vi "Select SubProtocol.vi"(7 "Set?":bool, 8 "error in (no error)":errorcluster, 11 "Connection.WS in":refnum<class "Connection.WS.lvclass">) -> (0 "error out":errorcluster, 3 "Connection.WS out":refnum<class "Connection.WS.lvclass">)   [LabVIEW 2013, in "Connection.WS_GOSPL.lvlib" / "Connection.WS.lvclass"]
uses:
  Connection.WS.lvclass
  Connection.WS.lvclass/Connection.WS.ctl
  Header Fields -- combo.ctl
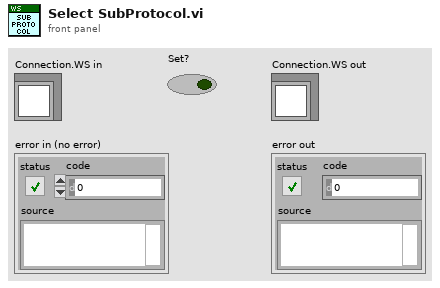
[diagram p1: front panel]
types:
  T1 = typedef "Connection.WS_GOSPL.lvlib/Connection.WS.lvclass/Header Fields -- combo.ctl" = string
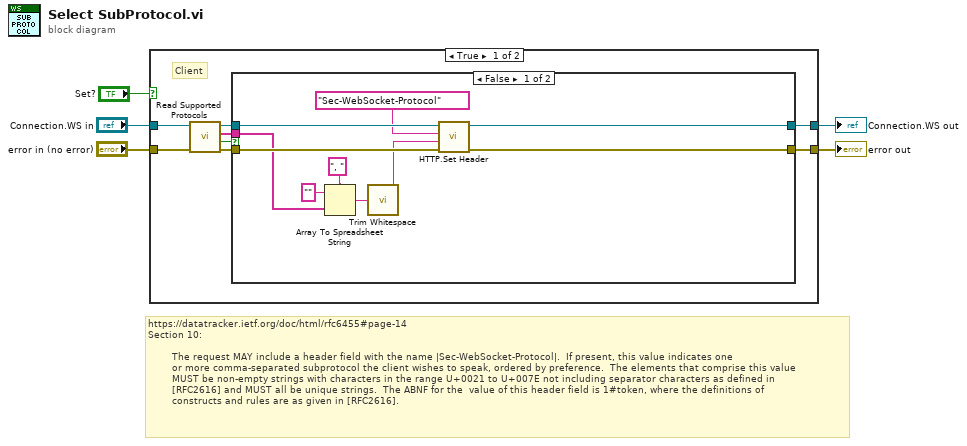
[diagram p0: block diagram]
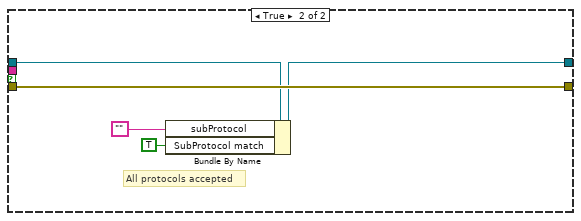
[diagram p2: hidden frame]
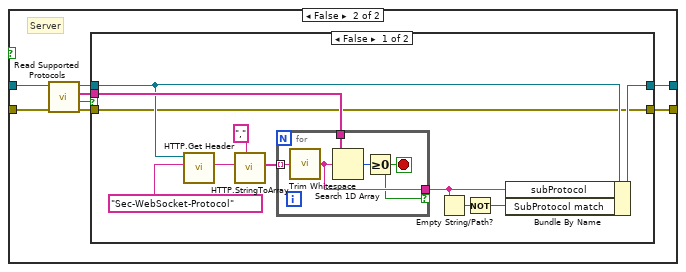
[diagram p3: hidden frame]
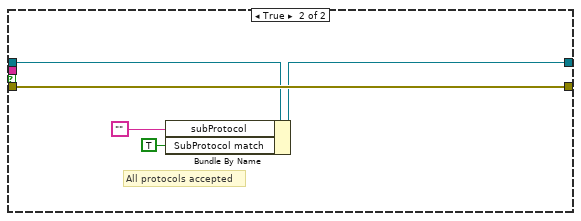
[diagram p4: hidden frame]
diagram:
  # "https://datatracker.ietf.org/doc/html/rfc6455#page-14\nSection 10:\n\n        The request MAY include a header field with the name |Sec-WebSocket-Protocol|.  If present, this value indicates one\n        or more comma-separated subprotocol the client wishes to speak, ordered by preference.  The elements that comprise this value\n        MUST be non-empty strings with characters in the range U+0021 to U+007E not including separator characters as defined in\n        [RFC2616] and MUST all be unique strings.  The ABNF for the  value of this header field is 1#token, where the definitions of\n        constructs and rules are as given in [RFC2616]."
  n1 = case shown="True" "Set?" {
    tunnel: [w11 w34] -> w5
    tunnel: [w10 w33] -> w4
    tunnel: "Connection.WS in" -> [w7 w30]
    tunnel: "error in (no error)" -> [w6 w29]
    frame True {
      # "Client"
      n2 = call "Read Supported Protocols.vi"("error in (no error)"=w6, "Connection.WS in"=w7) -> ("error out"=w12:errorcluster, "All?"=w8:bool, "Supported Protocols"=w13:string[], "Connection.WS out"=w9:refnum<class "Connection.WS.lvclass">)  [unwired: 6 in]
      n3 = case shown="False" w8 {
        tunnel: w9 -> [w23 w26]
        tunnel: [w22 w25] -> w10
        tunnel: [w20 w28] -> w11
        tunnel: w12 -> [w21 w28]
        tunnel: w13 -> [w18 _]
        frame False {
          n4 = Array To Spreadsheet String(delimiter (Tab)=", ", array=w18, 3:"" ("format string")) -> (spreadsheet string=w16:string)
          n5 = call <vilib>:"Trim Whitespace.vi"("string"=w16) -> ("trimmed string"=w14:string)  [unwired: 1 in]
          n6 = call "HTTP.Set Header.vi"("error in (no error)"=w21, "Value"=w14, "Header Name"=T1 "Sec-WebSocket-Protocol", "Connection.WS in"=w23) -> ("error out"=w20:errorcluster, "Connection.WS out"=w22:refnum<class "Connection.WS.lvclass">)  [unwired: 6 in]
        }
        frame True {
          # "All protocols accepted"
          n7 = Bundle By Name(cluster=w26, "subProtocol"="", "SubProtocol match"=TRUE) -> (w25:refnum<class "Connection.WS.lvclass">)
        }
      }
    }
    frame False {
      # "Server"
      n8 = call "Read Supported Protocols.vi"("error in (no error)"=w29, "Connection.WS in"=w30) -> ("error out"=w35:errorcluster, "All?"=w31:bool, "Supported Protocols"=w36:string[], "Connection.WS out"=w32:refnum<class "Connection.WS.lvclass">)  [unwired: 6 in]
      n9 = case shown="False" w31 {
        tunnel: w32 -> [w38 w55]
        tunnel: [w43 w54] -> w33
        tunnel: [w37 w57] -> w34
        tunnel: w35 -> [w37 w57]
        tunnel: w36 -> [w45 _]
        frame False {
          n10 = call "HTTP.Get Header.vi"("Header Name"=T1 "Sec-WebSocket-Protocol", "Connection.WS in"=w38) -> ("Value"=w44:string)  [unwired: 6 in, 3 out]
          n11 = call "HTTP.StringToArray.vi"("Separator"=",", "string"=w44) -> ("Array"=w46:string[])  [unwired: 9 in]
          n12 = for {
            tunnel: w46 -> [w52] mode=indexing
            tunnel: w45 -> [w50]
            tunnel: [w49] -> w42 if=w48
            stop <- w48 stop-if-true
            n13 = call <vilib>:"Trim Whitespace.vi"("string"=w52) -> ("trimmed string"=w49:string)  [unwired: 1 in]
            n14 = Search 1D Array(1D array=w50, element=w49) -> (index of element=w51:i32)  [unwired: 1 in]
            n15 = Greater Or Equal To 0?(x=w51) -> (x >= 0?=w48:bool)
          }
          n16 = Empty String/Path?(string/path=w42) -> (empty?=w41:bool)
          n17 = Not(x=w41) -> (.not. x?=w40:bool)
          n18 = Bundle By Name(cluster=w38, "subProtocol"=w42, "SubProtocol match"=w40) -> (w43:refnum<class "Connection.WS.lvclass">)
        }
        frame True {
          # "All protocols accepted"
          n19 = Bundle By Name(cluster=w55, "subProtocol"="", "SubProtocol match"=TRUE) -> (w54:refnum<class "Connection.WS.lvclass">)
        }
      }
    }
  }
  "error out" <- w5
  "Connection.WS out" <- w4
